vi "aptControl.vi"() -> (0 "Moving":bool, 3 "Current Position":sgl)   [LabVIEW 2014]
uses:
  <vilib>/DAQmx/write.llb/DAQmx Write (Digital 1D Bool 1Chan 1Samp).vi
  <vilib>/DAQmx/write.llb/DAQmx Write (Analog Wfm 1Chan NSamp).vi
  <vilib>/DAQmx/read.llb/DAQmx Read (Analog Wfm 1Chan NSamp).vi
  <vilib>/Analysis/baseanly.llb/Mean (DBL).vi
  <vilib>/DAQmx/miscellaneous.llb/DAQmx Fill In Error Info.vi
  <vilib>/Utility/file.llb/Write To Spreadsheet File (DBL).vi
  <vilib>/Utility/file.llb/Read From Spreadsheet File (DBL).vi
  <vilib>/gmath/NI_Gmath.lvlib
  <vilib>/Analysis/NI_AALBase.lvlib
panel:
  out "Power Min&Max":i32[](array[numeric])
  out "Setup":i32
  out "MirrorPosition":sgl
  out "SavePath":path
  out "MinPos":sgl
  out "MaxPos":sgl
  out "Scaner":string
  in  "Tab Control":enum32{"Control", "Curve", "Calibrate"}(tab)
  in  "Shutter":bool
  in  "Power (mW)":dbl format="%#.0f"
  in  "Possition (0:360)":dbl format="%#.2f"
  in  "Up":bool
  in  "Down":bool
  in  "Mirror\nOverride":bool
  in  "Galvo":bool=TRUE caption="AOD"
  in  "Lens":u16(ring)=10 items=["4X"=4, "10X"=10, "16X"=16, "20X"=20, "25X"=25, "40X"=40, "60X"=60]
  out "Error/Wait":bool
  in  "Home":bool
  in  "stop":bool
  in  "Auto":bool
  out "Calibration Used":string
  out "Curve":cluster{"all rows":dbl[], "all rows":dbl[]}(graph)
  out "Curve 2":cluster{i32[], i32[]}(graph)
  in  "Path":path=path "X:/2Pcalibration"
  in  "Start Calibration":bool
  in  "WaveLengths":dbl[](array[numeric])=[800.0, 890.0]
  out "Finished":bool
  in  "quit":bool
  out "Remaining\n min":dbl format="%#.2f"
  out "Acquiring":bool
  out "Waiting":bool
  out "Moving 2":bool
  in  "Repetitions":dbl=1.0
  in  "Step Size":dbl=4.0
  out "Current mW":dbl format="%#.0f"
  out "Old possition":sgl
  in  "AOD motor":refnum<k7>(container)
  in  "Target Position":dbl
  in  "Attenuator motor":refnum<k7>(container)
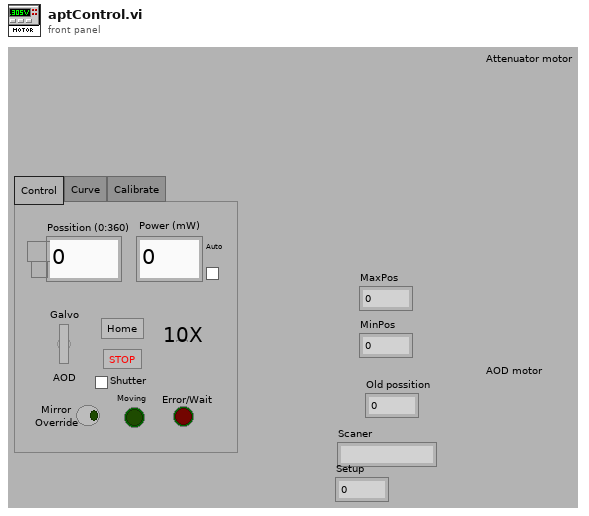
[diagram p1: front panel]
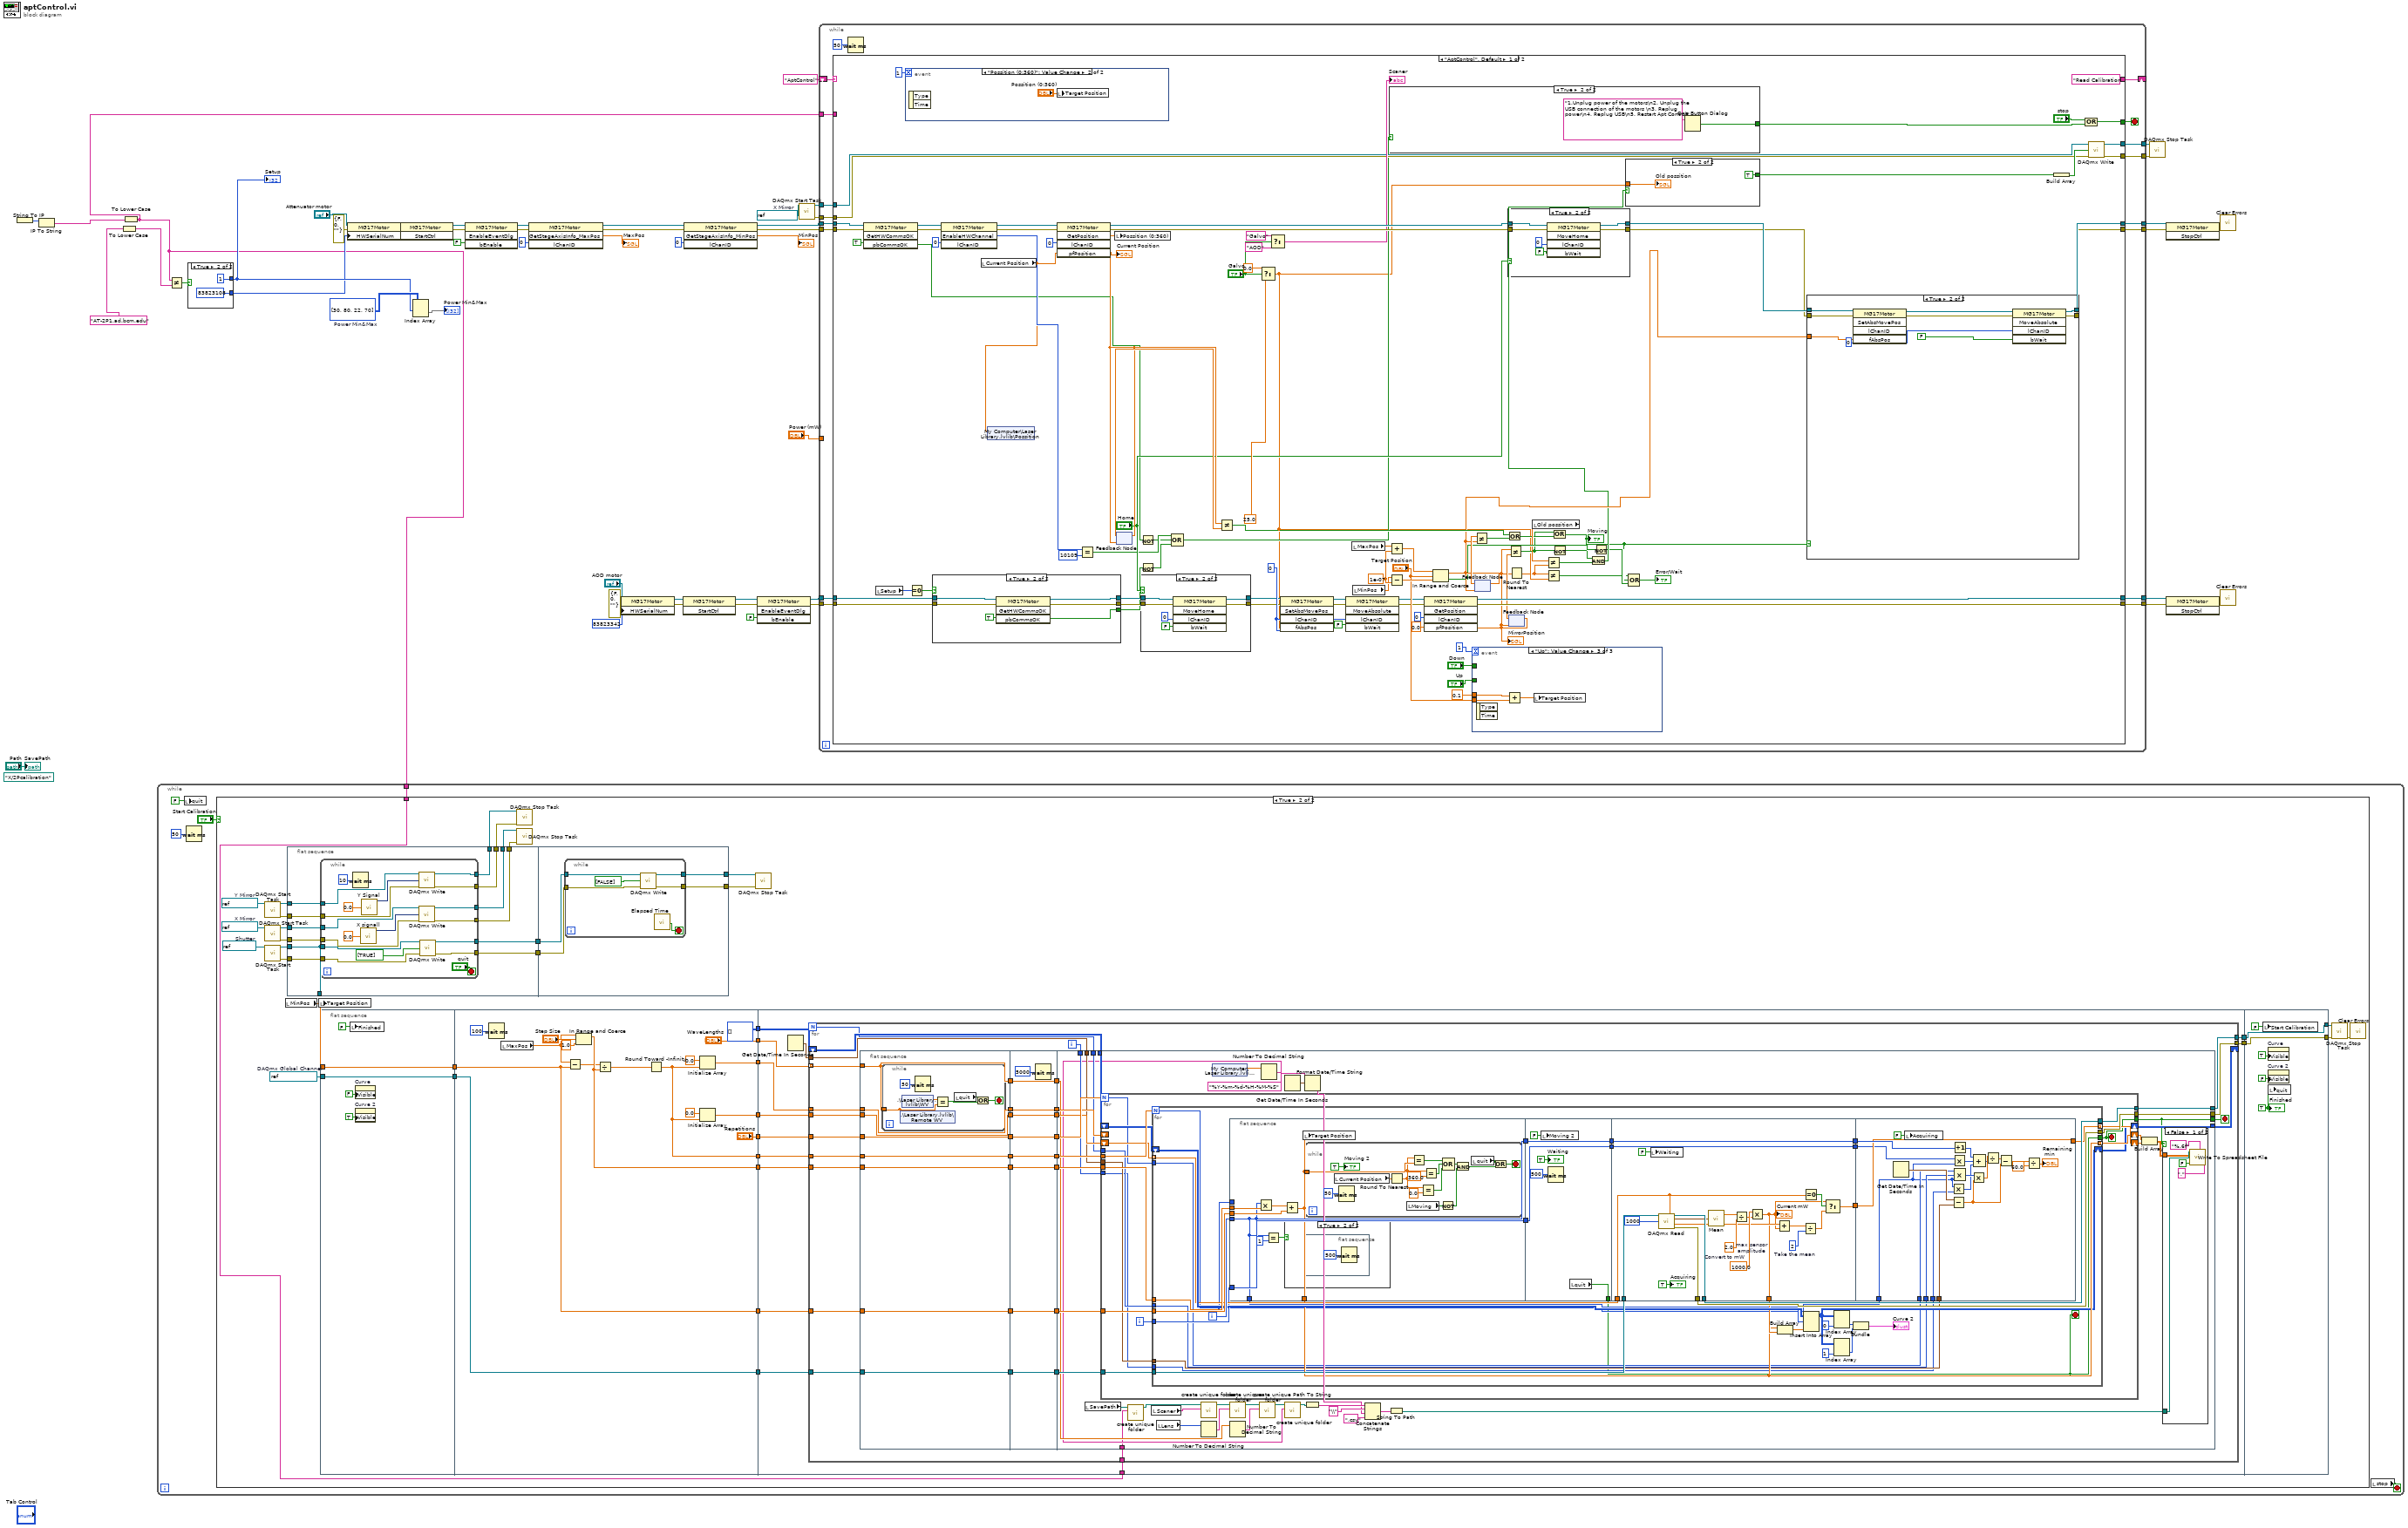
[diagram p0: block diagram]
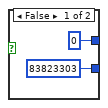
[diagram p2: hidden frame]
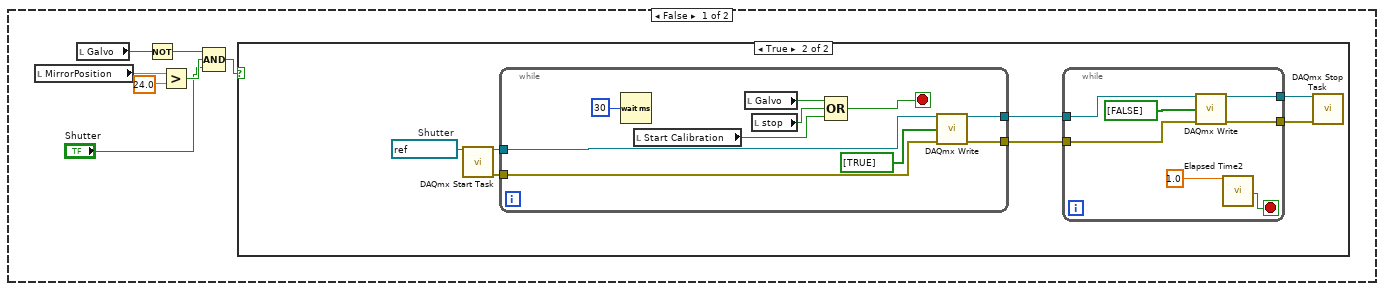
[diagram p3: hidden frame]
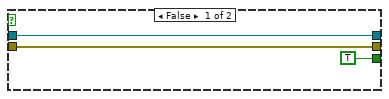
[diagram p7: hidden frame]
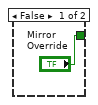
[diagram p9: hidden frame]
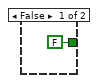
[diagram p10: hidden frame]
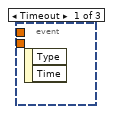
[diagram p11: hidden frame]
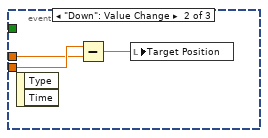
[diagram p12: hidden frame]
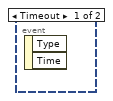
[diagram p13: hidden frame]
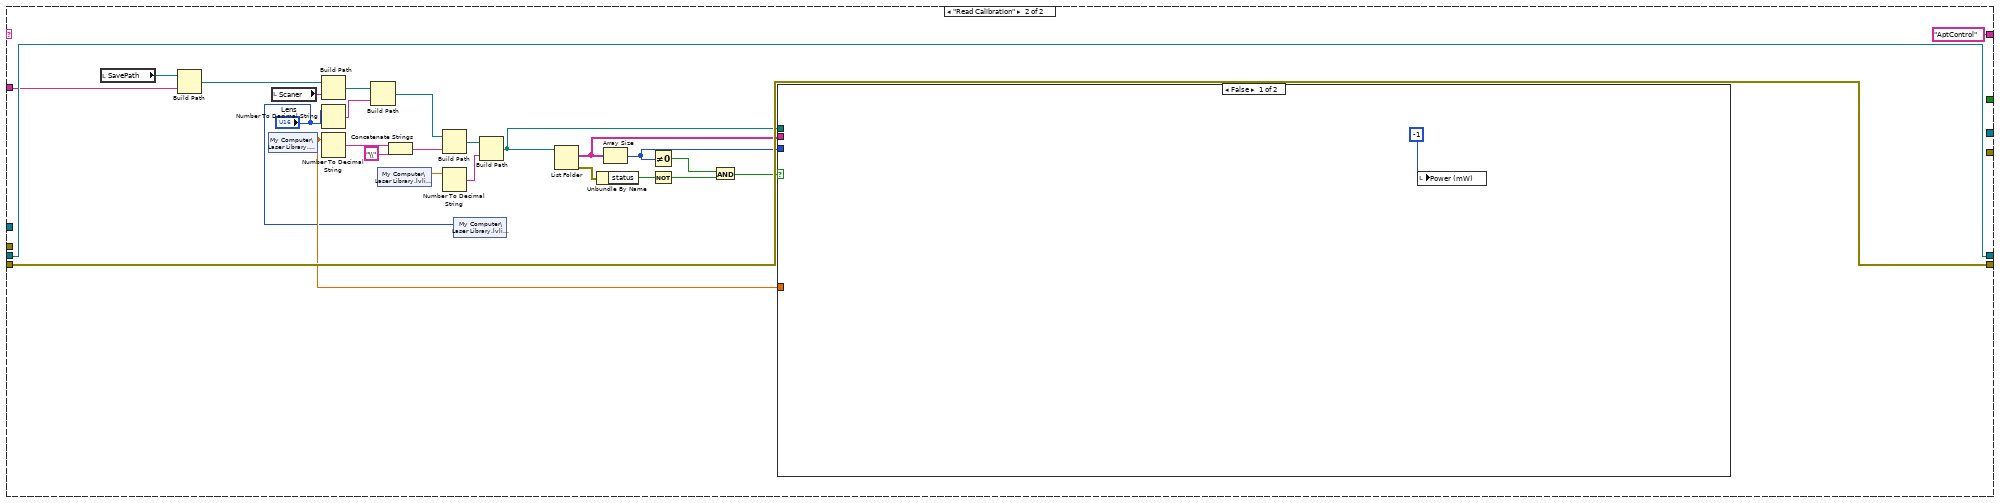
[diagram p16: hidden frame]
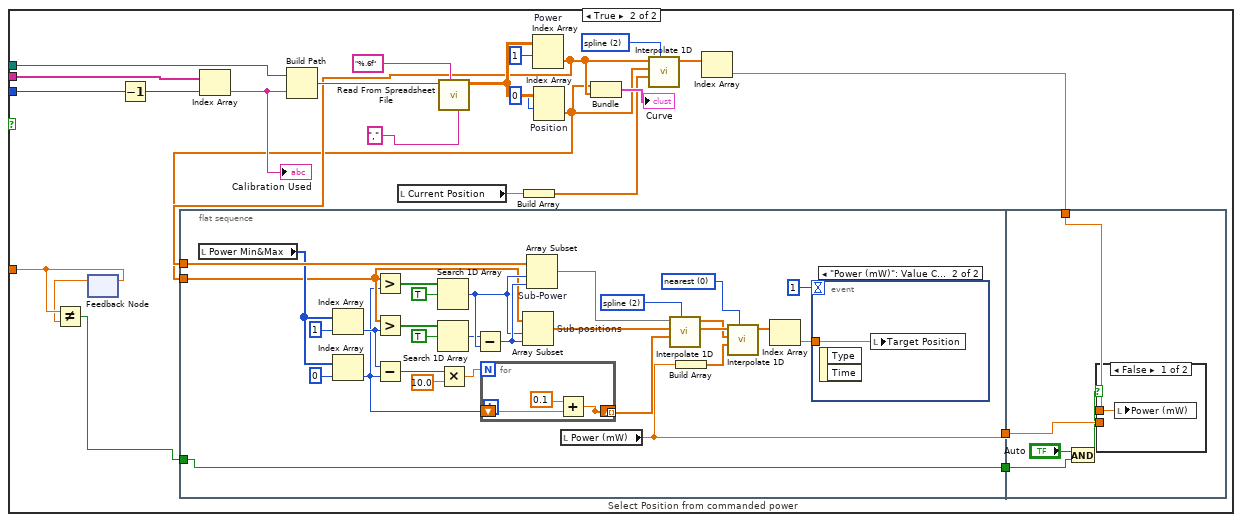
[diagram p17: hidden frame]
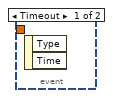
[diagram p18: hidden frame]
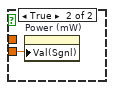
[diagram p19: hidden frame]
diagram:
  w11 = i32[][] [[30, 80], [22, 70]]  # Power Min&Max
  (unwired) path "X:/2Pcalibration"
  w20 = refnum<k21> "FlipMirror"  # X Mirror
  n1 = String To IP() -> (0:w8:u32)  [unwired: 1 in]
  n2 = IP To String(2:w8) -> (0:w4:string)  [unwired: 1 in]
  n3 = To Lower Case(string="AT-2P1.ad.bcm.edu") -> (all lower case string=w2:string)
  n4 = To Lower Case(string=w4) -> (all lower case string=w3:string)
  n5 = while {
    tunnel: w3 -> [w52]
    stop <- w55 stop-if-true
    n6 = local write "quit"(FALSE) -> ()
    n7 = Wait (ms)(milliseconds to wait=u32 50) -> ()  [unwired: 1 out]
    n8 = case shown="True" "Start Calibration" {
      tunnel: w52 -> [_ w88]
      frame False {
        n9 = local read "MirrorPosition"() -> (w63:sgl)
        n10 = local read "Galvo"() -> (w61:bool)
        n11 = Not(x=w61) -> (.not. x?=w62:bool)
        n12 = Greater?(x=w63, y=sgl 24.0) -> (0:w60:bool)
        n13 = Compound Arithmetic op=AND(w62, w60, "Shutter") -> (w58:bool)
        n14 = case shown="True" w58 {
          frame False {
          }
          frame True {
            w70 = refnum<k21> "Shutter"  # Shutter
            n15 = call <vilib>:"DAQmx Start Task.vi"("task/channels in"=w70) -> ("task out"=w69:refnum<k21>, "error out"=w68:errorcluster)  [unwired: 13 in]
            n16 = while {
              tunnel: w69 -> [w86]
              tunnel: w68 -> [w85]
              tunnel: [w84] -> w67
              tunnel: [w83] -> w66
              stop <- w80 stop-if-true
              n17 = Wait (ms)(milliseconds to wait=u32 30) -> ()  [unwired: 1 out]
              n18 = local read "Start Calibration"() -> (w81:bool)
              n19 = local read "Galvo"() -> (w78:bool)
              n20 = local read "stop"() -> (w82:bool)
              n21 = Compound Arithmetic op=OR(w78, w82, w81) -> (w80:bool)
              n22 = call-poly <vilib>:"DAQmx Write.vi"("task/channels in"=w86, "data"=bool[] [TRUE], "error in"=w85) -> ("task out"=w84:refnum<k21>, "error out"=w83:errorcluster)  [unwired: 10 in, 1 out]
            }
            n23 = while {
              tunnel: w67 -> [w77]
              tunnel: w66 -> [w76]
              tunnel: [w75] -> w65
              tunnel: [w74] -> w64
              stop <- w72 stop-if-true
              n24 = call-poly <vilib>:"DAQmx Write.vi"("task/channels in"=w77, "data"=bool[] [FALSE], "error in"=w76) -> ("task out"=w75:refnum<k21>, "error out"=w74:errorcluster)  [unwired: 10 in, 1 out]
              n25 = call "Elapsed Time2"("Time Target (s)"=1.0) -> ("Time has Elapsed"=w72:bool)  [unwired: 11 in, 7 out]
            }
            n26 = call <vilib>:"DAQmx Stop Task.vi"("task/channels in"=w65, "error in"=w64) -> ()  [unwired: 12 in, 2 out]
          }
        }
      }
      frame True {
        w96 = refnum<k21> "Y Mirror"  # Y Mirror
        w97 = refnum<k21> "X Mirror"  # X Mirror
        w98 = refnum<k21> "Shutter"  # Shutter
        w105 = refnum<k21> "PowerMeter"  # DAQmx Global Channel
        n27 = call <vilib>:"DAQmx Start Task.vi"("task/channels in"=w96) -> ("task out"=w95:refnum<k21>, "error out"=w90:errorcluster)  [unwired: 13 in]
        n28 = call <vilib>:"DAQmx Start Task.vi"("task/channels in"=w97) -> ("task out"=w93:refnum<k21>, "error out"=w91:errorcluster)  [unwired: 13 in]
        n29 = call <vilib>:"DAQmx Start Task.vi"("task/channels in"=w98) -> ("task out"=w94:refnum<k21>, "error out"=w92:errorcluster)  [unwired: 13 in]
        n30 = local read "MinPos"() -> (w89:sgl)
        n31 = flat-sequence {
          tunnel: [w127] -> _
          tunnel: w93 -> [w135]
          tunnel: [w134] -> w110
          tunnel: [w133] -> w109
          tunnel: [w132] -> w102
          tunnel: [w131] -> w101
          tunnel: [w130] -> w100
          tunnel: [w129] -> w99
          tunnel: w95 -> [w128]
          tunnel: w94 -> [w127]
          tunnel: w92 -> [w126]
          tunnel: w91 -> [w125]
          tunnel: w90 -> [w124]
          tunnel: w110 -> [w158]
          tunnel: [w157] -> w104
          tunnel: [w156] -> w103
          tunnel: w109 -> [w155]
          frame #0 {
            n32 = while {
              tunnel: w127 -> [w149]
              tunnel: w135 -> [w151]
              tunnel: w128 -> [w150]
              tunnel: [w147] -> w134
              tunnel: [w146] -> w133
              tunnel: [w143] -> w132
              tunnel: [w142] -> w131
              tunnel: [w141] -> w130
              tunnel: [w140] -> w129
              tunnel: w126 -> [w139]
              tunnel: w125 -> [w138]
              tunnel: w124 -> [w137]
              stop <- "quit" stop-if-true
              n33 = Wait (ms)(milliseconds to wait=u32 10) -> ()  [unwired: 1 out]
              n34 = call "X signall"("Amplitude"=0.0) -> ("Sine"=w145:dynamicdata)  [unwired: 13 in, 1 out]
              n35 = call "Y Signal"("Amplitude"=0.0) -> ("Sine"=w144:dynamicdata)  [unwired: 13 in, 1 out]
              n36 = call-poly <vilib>:"DAQmx Write.vi"("task/channels in"=w150, "data"=w144, "error in"=w137) -> ("task out"=w141:refnum<k21>, "error out"=w140:errorcluster)  [unwired: 10 in, 1 out]
              n37 = call-poly <vilib>:"DAQmx Write.vi"("task/channels in"=w151, "data"=w145, "error in"=w138) -> ("task out"=w143:refnum<k21>, "error out"=w142:errorcluster)  [unwired: 10 in, 1 out]
              n38 = call-poly <vilib>:"DAQmx Write.vi"("task/channels in"=w149, "data"=bool[] [TRUE], "error in"=w139) -> ("task out"=w147:refnum<k21>, "error out"=w146:errorcluster)  [unwired: 10 in, 1 out]
            }
          }
          frame #1 {
            n39 = while {
              tunnel: w158 -> [w163]
              tunnel: [w161] -> w157
              tunnel: [w160] -> w156
              tunnel: w155 -> [w159]
              stop <- w164 stop-if-true
              n40 = call-poly <vilib>:"DAQmx Write.vi"("task/channels in"=w163, "data"=bool[] [FALSE], "error in"=w159) -> ("task out"=w161:refnum<k21>, "error out"=w160:errorcluster)  [unwired: 10 in, 1 out]
              n41 = call "Elapsed Time"() -> ("Time has Elapsed"=w164:bool)  [unwired: 12 in, 7 out]
            }
          }
        }
        n42 = local write "Target Position"(w89) -> ()
        n43 = flat-sequence {
          tunnel: w105 -> [w168]
          tunnel: w89 -> [w169]
          tunnel: [w169] -> w123
          tunnel: [w168] -> w122
          tunnel: [w184] -> w121
          tunnel: ["Repetitions"] -> w120
          tunnel: [w183] -> w119
          tunnel: [w186] -> w118
          tunnel: [w182] -> w117
          tunnel: [w181] -> w116
          tunnel: [i32[][] []] -> w115
          tunnel: ["WaveLengths"] -> w114
          tunnel: [w180] -> w113
          tunnel: w123 -> [w184]
          tunnel: w122 -> [w186]
          tunnel: w121 -> [w199]
          tunnel: w120 -> [w198]
          tunnel: w119 -> [w197]
          tunnel: w118 -> [w196]
          tunnel: w117 -> [w194]
          tunnel: w116 -> [w193]
          tunnel: w115 -> [w191]
          tunnel: w114 -> [w192]
          tunnel: w113 -> [w195]
          tunnel: [w190] -> w112
          tunnel: [w189] -> w111
          tunnel: w88 -> [w187]
          tunnel: [w427] -> w106
          tunnel: [w428] -> w107
          tunnel: w112 -> [w428]
          tunnel: w111 -> [w427]
          frame #0 {
            n44 = local write "Finished"(FALSE ("Finished")) -> ()
            n45 = property on="Curve" class="XYGraph (strict)"("Visible"=FALSE) -> ()  [unwired: 2 in, 2 out]
            n46 = property on="Curve 2" class="XYGraph (strict)"("Visible"=TRUE) -> ()  [unwired: 2 in, 2 out]
          }
          frame #1 {
            n47 = Wait (ms)(milliseconds to wait=u32 100) -> ()  [unwired: 1 out]
            n48 = local read "MaxPos"() -> (w170:sgl)
            n49 = Subtract(x=w170, y=w184) -> (x-y=w175:sgl)
            n50 = In Range and Coerce(upper limit=w170, x="Step Size", lower limit=1.0) -> (coerced(x)=w183:dbl)  [unwired: 1 out]
            n51 = Divide(x=w175, y=w183) -> (x/y=w176:dbl)
            n52 = Round Toward -Infinity(1:w176) -> (0:w182:dbl)
            n53 = Initialize Array(0.0 ("element"), w182) -> (w181:dbl[])
            n54 = Initialize Array(0.0 ("element"), w182) -> (w180:dbl[])
          }
          frame #2 {
            n55 = Get Date/Time In Seconds() -> (seconds since 1Jan1904=w188:timestamp)
            n56 = for {
              N -> [w203]
              tunnel: w199 -> [w232]
              tunnel: w198 -> [w231]
              tunnel: w197 -> [w230]
              tunnel: w196 -> [w229]
              tunnel: [w228] -> w190
              tunnel: [w227] -> w189
              tunnel: w195 -> [w226]
              tunnel: w194 -> [w225]
              tunnel: w193 -> [w224]
              tunnel: w192 -> [w223] mode=indexing
              shift-right: [w205] -> _
              shift-left: w191 -> [w206]
              tunnel: w188 -> [w204]
              tunnel: w187 -> [w200]
              i -> [w202]
              stop <- w201 stop-if-true
              n57 = flat-sequence {
                tunnel: w223 -> [w233]
                tunnel: w224 -> [w234]
                tunnel: w225 -> [w235]
                tunnel: w226 -> [w236]
                tunnel: w229 -> [w237]
                tunnel: w230 -> [w238]
                tunnel: w231 -> [w239]
                tunnel: w232 -> [w240]
                tunnel: [w240] -> w222
                tunnel: [w239] -> w220
                tunnel: [w238] -> w218
                tunnel: [w237] -> w216
                tunnel: [w236] -> w214
                tunnel: [w235] -> w212
                tunnel: [w234] -> w210
                tunnel: [w233] -> w208
                tunnel: w222 -> [w255]
                tunnel: [w255] -> w221
                tunnel: w220 -> [w254]
                tunnel: [w254] -> w219
                tunnel: w218 -> [w253]
                tunnel: [w253] -> w217
                tunnel: w216 -> [w252]
                tunnel: [w252] -> w215
                tunnel: w214 -> [w251]
                tunnel: [w251] -> w213
                tunnel: w212 -> [w250]
                tunnel: [w250] -> w211
                tunnel: w210 -> [w249]
                tunnel: [w249] -> w209
                tunnel: w208 -> [w248]
                tunnel: [w248] -> w207
                tunnel: [w293] -> w205
                tunnel: [w294] -> w227
                tunnel: [w295] -> w228
                tunnel: w202 -> [w267]
                tunnel: w203 -> [w268]
                tunnel: w204 -> [w269]
                tunnel: w206 -> [w270]
                tunnel: w207 -> [w271]
                tunnel: w209 -> [w286]
                tunnel: w211 -> [w287]
                tunnel: w213 -> [w288]
                tunnel: w215 -> [w289]
                tunnel: w217 -> [w290]
                tunnel: w219 -> [w291]
                tunnel: w221 -> [w292]
                tunnel: [w258] -> w201
                tunnel: w200 -> [w256]
                frame #0 {
                  n58 = while {
                    tunnel: w233 -> [w245]
                    stop <- w241 stop-if-true
                    n59 = shared-variable ".\\Laser Library.lvlib\\Remote WV"(w245) -> ()  [unwired: 1 in, 1 out]
                    n60 = shared-variable ".\\Laser Library.lvlib\\WV"() -> (w244:dbl)  [unwired: 1 in, 1 out]
                    n61 = Wait (ms)(milliseconds to wait=u32 50) -> ()  [unwired: 1 out]
                    n62 = Equal?(x=w244, y=w245) -> (x = y?=w242:bool)
                    n63 = local read "quit"() -> (w243:bool)
                    n64 = Or(x=w243, y=w242) -> (x .or. y?=w241:bool)
                  }
                }
                frame #1 {
                  n65 = Wait (ms)(milliseconds to wait=u32 5000) -> ()  [unwired: 1 out]
                }
                frame #2 {
                  n66 = local read "SavePath"() -> (w257:path)
                  n67 = for {
                    N: w291 -> [w303]
                    tunnel: w287 -> [w317]
                    tunnel: w292 -> [w316]
                    tunnel: w290 -> [w315]
                    tunnel: w289 -> [w314]
                    tunnel: [w313] -> w295
                    tunnel: [w312] -> w294
                    shift-right: [w311] -> w273
                    shift-left: w288 -> [w309]
                    shift-right: [w310] -> w274
                    shift-left: w286 -> [_]
                    shift-right: [w308] -> w293
                    shift-left: w270 -> [w307]
                    tunnel: w269 -> [w305]
                    tunnel: w268 -> [w304]
                    tunnel: w267 -> [w302]
                    tunnel: [w301] -> w258
                    i -> [w306]
                    stop <- w301 stop-if-true
                    n68 = for {
                      N: w317 -> [w321]
                      tunnel: w316 -> [w350]
                      tunnel: w315 -> [w349]
                      tunnel: w314 -> [w347]
                      tunnel: [w346] -> w313
                      tunnel: [w345] -> w312
                      tunnel: [w320] -> w311 mode=indexing
                      tunnel: w309 -> [w342] mode=indexing
                      tunnel: [w338] -> w310 mode=indexing
                      shift-right: [w335] -> w308
                      shift-left: w307 -> [w343]
                      tunnel: w306 -> [w332]
                      tunnel: w305 -> [w331]
                      tunnel: w304 -> [w330]
                      tunnel: w303 -> [w329]
                      tunnel: w302 -> [w328]
                      tunnel: [w319] -> w301
                      i -> [w348]
                      stop <- w319 stop-if-true
                      n69 = flat-sequence {
                        tunnel: w348 -> [w354]
                        tunnel: w349 -> [w358]
                        tunnel: w350 -> [w355]
                        tunnel: [w351] -> w338
                        tunnel: [w354] -> w339
                        tunnel: w332 -> [w357]
                        tunnel: [w357] -> w325
                        tunnel: [w354] -> w322
                        tunnel: w321 -> [_]
                        tunnel: [w380] -> w326
                        tunnel: w325 -> [w380]
                        tunnel: [w379] -> w323
                        tunnel: w322 -> [w379]
                        tunnel: [w376] -> w319
                        tunnel: w347 -> [w401]
                        tunnel: [w400] -> w346
                        tunnel: [w399] -> w345
                        tunnel: w342 -> [w385]
                        tunnel: [w393] -> w344
                        tunnel: [w382] -> w341
                        tunnel: [w387] -> w327
                        tunnel: w326 -> [w387]
                        tunnel: [w386] -> w324
                        tunnel: w323 -> [w386]
                        tunnel: w344 -> [w416]
                        tunnel: w331 -> [w421]
                        tunnel: w330 -> [w420]
                        tunnel: w329 -> [w419]
                        tunnel: w321 -> [w408]
                        tunnel: w328 -> [w409]
                        tunnel: w327 -> [w410]
                        tunnel: w324 -> [w418]
                        tunnel: [w416] -> w320
                        frame #0 {
                          n70 = Multiply(x=w354, y=w358) -> (x*y=w356:dbl)
                          n71 = Equal?(x=w354, y=1) -> (x = y?=w353:bool)
                          n72 = Add(x=w356, y=w355) -> (x+y=w351:dbl)
                          n73 = case shown="True" w353 {
                            frame False {
                            }
                            frame True {
                              n74 = flat-sequence {
                                frame #0 {
                                n75 = Wait (ms)(milliseconds to wait=u32 500) -> ()  [unwired: 1 out]
                                }
                              }
                            }
                          }
                          n76 = local write "Target Position"(w351) -> ()
                          n77 = while {
                            tunnel: w351 -> [w374]
                            stop <- w361 stop-if-true
                            n78 = local read "Current Position"() -> (w363:sgl)
                            n79 = Wait (ms)(milliseconds to wait=u32 50) -> ()  [unwired: 1 out]
                            n80 = Round To Nearest(number=w363) -> (nearest integer value=w368:sgl)
                            n81 = local read "Moving"() -> (w364:bool)
                            n82 = Equal?(x=w368, y=w374) -> (x = y?=w372:bool)
                            n83 = Equal?(x=w368, y=0.0) -> (x = y?=w369:bool)
                            n84 = Equal?(x=w368, y=360.0) -> (x = y?=w370:bool)
                            n85 = Not(x=w364) -> (.not. x?=w373:bool)
                            n86 = Compound Arithmetic op=OR(w372, w370, w369) -> (w371:bool)
                            n87 = And(x=w371, y=w373) -> (x .and. y?=w362:bool)
                            n88 = local read "quit"() -> (w360:bool)
                            n89 = Or(x=w360, y=w362) -> (x .or. y?=w361:bool)
                            "Moving 2" <- TRUE
                          }
                        }
                        frame #1 {
                          n90 = local write "Moving 2"(FALSE) -> ()
                          n91 = Wait (ms)(milliseconds to wait=u32 500) -> ()  [unwired: 1 out]
                          n92 = local read "quit"() -> (w376:bool)
                          "Waiting" <- TRUE
                        }
                        frame #2 {
                          w388 = 2.0  # max sensor  amplitude
                          w390 = 1000.0  # Convert to mW
                          w396 = 2  # Take the mean
                          n93 = local write "Waiting"(FALSE) -> ()
                          n94 = call-poly <vilib>:"DAQmx Read.vi"("task/channels in"=w401, "number of samples per channel"=1000) -> ("task out"=w400:refnum<k21>, "data"=w391:waveform(dbl), "error out"=w399:errorcluster)  [unwired: 1 in, 10 out]
                          n95 = call-poly <vilib>:"Mean.vi"("X"=w391) -> ("mean"=w392:dbl)  [unwired: 1 out]
                          n96 = Divide(x=w392, y=w388) -> (x/y=w389:dbl)
                          n97 = Multiply(x=w390, y=w389) -> (x*y=w382:dbl)
                          "Current mW" <- w382
                          n98 = Add(x=w385, y=w382) -> (x+y=w395:dbl)
                          n99 = Divide(x=w395, y=w396) -> (x/y=w394:dbl)
                          n100 = Equal To 0?(x=w385) -> (x = 0?=w397:bool)
                          n101 = Select(t=w382, s=w397, f=w394) -> (s? t:f=w393:dbl)
                          "Acquiring" <- TRUE ("Acquiring")
                        }
                        frame #3 {
                          n102 = Get Date/Time In Seconds() -> (seconds since 1Jan1904=w422:timestamp)
                          n103 = local write "Acquiring"(FALSE ("Acquiring")) -> ()
                          n104 = Multiply(x=w408, y=w409) -> (x*y=w405:i32)
                          n105 = Subtract(x=w422, y=w421) -> (x-y=w413:dbl)
                          n106 = Multiply(x=w410, y=w408) -> (x*y=w406:i32)
                          n107 = Increment(x=w418) -> (x+1=w407:i32)
                          n108 = Compound Arithmetic op=MULTIPLY(w419, w420, w408) -> (w415:i32)
                          n109 = Multiply(x=w415, y=w413) -> (x*y=w414:dbl)
                          n110 = Compound Arithmetic op=ADD(w407, w406, w405) -> (w404:i32)
                          n111 = Divide(x=w414, y=w404) -> (x/y=w412:dbl)
                          n112 = Subtract(x=w412, y=w413) -> (x-y=w411:dbl)
                          n113 = Divide(x=w411, y=60.0) -> (x/y=→"Remaining\n min":dbl)
                        }
                      }
                      n114 = Build Array(w338, w341) -> (w340:dbl[])
                      n115 = Insert Into Array(array=w343, index (row)=w339, new element=w340) -> (w335:i32[][])  [unwired: 1 in]
                      n116 = Index Array(array=w335, index (col)=0 ("index")) -> (element=w336:i32[])  [unwired: 1 in]
                      n117 = Index Array(array=w335, index (col)=1 ("index")) -> (element=w333:i32[])  [unwired: 1 in]
                      n118 = Bundle(w336, w333) -> (→"Curve 2":cluster{i32[], i32[]})  [unwired: 1 in]
                    }
                  }
                  n119 = call "create unique folder.vi"("string"=w256, "path 2"=w257) -> ("path"=w266:path)  [unwired: 9 in]
                  n120 = local read "Scaner"() -> (w259:string)
                  n121 = local read "Lens"() -> (w260:u16)
                  n122 = call "create unique folder.vi"("string"=w259, "path 2"=w266) -> ("path"=w265:path)  [unwired: 9 in]
                  n123 = Number To Decimal String(number=w260) -> (decimal integer string=w275:string)  [unwired: 1 in]
                  n124 = shared-variable "My Computer\\Laser Library.lvlib\\GDD"() -> (w264:dbl)  [unwired: 1 in, 1 out]
                  n125 = call "create unique folder.vi"("string"=w275, "path 2"=w265) -> ("path"=w276:path)  [unwired: 9 in]
                  n126 = Number To Decimal String(number=w271) -> (decimal integer string=w283:string)  [unwired: 1 in]
                  n127 = call "create unique folder.vi"("string"=w283, "path 2"=w276) -> ("path"=w263:path)  [unwired: 9 in]
                  n128 = Number To Decimal String(number=w264) -> (decimal integer string=w261:string)  [unwired: 1 in]
                  n129 = Get Date/Time In Seconds() -> (seconds since 1Jan1904=w285:timestamp)
                  n130 = call "create unique folder.vi"("string"=w261, "path 2"=w263) -> ("path"=w262:path)  [unwired: 9 in]
                  n131 = Path To String(path=w262) -> (string=w282:string)
                  n132 = Format Date/Time String(time format string (%c)="%Y-%m-%d-%H-%M-%S", seconds (now)=w285) -> (date/time string=w280:string)  [unwired: 1 in]
                  n133 = Concatenate Strings(w282, "\\" ("string"), w280, ".csv" ("string")) -> (w279:string)
                  n134 = String To Path(string=w279) -> (path=w278:path)
                  n135 = Build Array(w274, w273) -> (w272:dbl[][])
                  n136 = case shown="False" w258 {
                    tunnel: w278 -> [w297 _]
                    tunnel: w272 -> [w296 _]
                    frame False {
                      n137 = call-poly <vilib>:"Write To Spreadsheet File.vi"("delimiter (\\t)"="," ("delimiter (\\t)"), "format (%.3f)"="%.6f", "append to file? (new file:F)"=FALSE, "2D data"=w296, "file path (dialog if empty)"=w297) -> ()  [unwired: 2 in, 2 out]
                    }
                    frame True {
                    }
                  }
                }
              }
            }
          }
          frame #3 {
            w426 = TRUE ("Finished")
            n138 = local write "Start Calibration"(FALSE) -> ()
            n139 = property on="Curve" class="XYGraph (strict)"("Visible"=TRUE) -> ()  [unwired: 2 in, 2 out]
            n140 = property on="Curve 2" class="XYGraph (strict)"("Visible"=FALSE) -> ()  [unwired: 2 in, 2 out]
            n141 = local write "quit"(w426) -> ()
            "Finished" <- w426
          }
        }
        n142 = call <vilib>:"DAQmx Stop Task.vi"("task/channels in"=w100, "error in"=w99) -> ()  [unwired: 12 in, 2 out]
        n143 = call <vilib>:"DAQmx Stop Task.vi"("task/channels in"=w102, "error in"=w101) -> ()  [unwired: 12 in, 2 out]
        n144 = call <vilib>:"DAQmx Stop Task.vi"("task/channels in"=w104, "error in"=w103) -> ()  [unwired: 12 in, 2 out]
        n145 = call <vilib>:"DAQmx Stop Task.vi"("task/channels in"=w107, "error in"=w106) -> ("error out"=w108:errorcluster)  [unwired: 13 out]
        n146 = call <vilib>:"Clear Errors.vi"("error in (no error)"=w108) -> ()  [unwired: 5 in, 2 out]
      }
    }
    n147 = local read "stop"() -> (w55:bool)
  }
  n148 = Not Equal?(x=w3, y=w2) -> (x != y?=w7:bool)
  n149 = case shown="True" w7 {
    tunnel: [0 1] -> w6
    tunnel: [83823303 83823108] -> w5
    frame False {
    }
    frame True {
    }
  }
  "Setup" <- w6
  n150 = property class="MG17Motor"(reference="Attenuator motor", error in=errorcluster {"status"=FALSE, "code"=0, "source"=""} ("error in (no error)"), "HWSerialNum"=w5) -> (reference out=w50:refnum<k7>, error out=w49:errorcluster)
  n151 = invoke class="MG17Motor" method="StartCtrl"(reference=w50, error in=w49) -> (reference out=w38:refnum<k7>, error out=w37:errorcluster)  [unwired: 1 in, 1 out]
  n152 = Index Array(array=w11, index (row)=w6) -> (element=→"Power Min&Max":i32[])  [unwired: 1 in]
  n153 = invoke class="MG17Motor" method="EnableEventDlg"(reference=w38, error in=w37, "bEnable"=FALSE) -> (reference out=w36:refnum<k7>, error out=w35:errorcluster)  [unwired: 1 in, 2 out]
  n154 = invoke class="MG17Motor" method="GetStageAxisInfo_MaxPos"(reference=w36, error in=w35, "lChanID"=0) -> (reference out=w41:refnum<k7>, error out=w40:errorcluster, "GetStageAxisInfo_MaxPos"=→"MaxPos":sgl)  [unwired: 1 in, 1 out]
  n155 = property class="MG17Motor"(reference="AOD motor", error in=errorcluster {"status"=FALSE, "code"=0, "source"=""} ("error in (no error)"), "HWSerialNum"=83823342) -> (reference out=w30:refnum<k7>, error out=w31:errorcluster)
  n156 = invoke class="MG17Motor" method="StartCtrl"(reference=w30, error in=w31) -> (reference out=w33:refnum<k7>, error out=w34:errorcluster)  [unwired: 1 in, 1 out]
  n157 = invoke class="MG17Motor" method="GetStageAxisInfo_MinPos"(reference=w41, error in=w40, "lChanID"=0) -> (reference out=w48:refnum<k7>, error out=w43:errorcluster, "GetStageAxisInfo_MinPos"=→"MinPos":sgl)  [unwired: 1 in, 1 out]
  n158 = invoke class="MG17Motor" method="EnableEventDlg"(reference=w33, error in=w34, "bEnable"=FALSE) -> (reference out=w28:refnum<k7>, error out=w23:errorcluster)  [unwired: 1 in, 2 out]
  n159 = call <vilib>:"DAQmx Start Task.vi"("task/channels in"=w20) -> ("task out"=w17:refnum<k21>, "error out"=w16:errorcluster)  [unwired: 13 in]
  n160 = while {
    tunnel: w48 -> [w449]
    tunnel: [w446] -> w46
    tunnel: [w447] -> w45
    tunnel: w43 -> [w445]
    shift-right: [w442] -> _
    shift-left: "AptControl" -> [w443]
    tunnel: w3 -> [w441]
    tunnel: w28 -> [w440]
    tunnel: [w439] -> w25
    tunnel: [w438] -> w24
    tunnel: w23 -> [w437]
    tunnel: [w436] -> w19
    tunnel: [w435] -> w18
    tunnel: w17 -> [w434]
    tunnel: w16 -> [w433]
    tunnel: "Power (mW)" -> [_]
    stop <- w444 stop-if-true
    n161 = case shown="\"AptControl\", Default" w443 {
      tunnel: w449 -> [w475 w614]
      tunnel: [w530 w614] -> w447
      tunnel: [w529 w613] -> w446
      tunnel: w445 -> [w473 w613]
      tunnel: [w523 _] -> w444
      tunnel: ["Read Calibration" "AptControl"] -> w442
      tunnel: w441 -> [_ w610]
      tunnel: w440 -> [w471 _]
      tunnel: [w501 _] -> w439
      tunnel: [w500 _] -> w438
      tunnel: w437 -> [w469 _]
      tunnel: [w482 _] -> w436
      tunnel: [w481 _] -> w435
      tunnel: w434 -> [w480 _]
      tunnel: w433 -> [w479 _]
      frame "AptControl", Default {
        w509 = 0 ("lChanID")
        w532 = 1e-07
        n162 = invoke class="MG17Motor" method="GetHWCommsOK"(reference=w475, error in=w473, "pbCommsOK"=TRUE) -> (reference out=w474:refnum<k7>, error out=w472:errorcluster, "pbCommsOK"=w463:bool)  [unwired: 1 in, 1 out]
        n163 = local read "Setup"() -> (w452:i32)
        n164 = event shown="[1] \"Possition (0:360)\": Value Change" {
          selector: _ -> [_ _]
          dyn-events: _ -> [_ _]
          timeout: 1 -> [_ _]
          event Timeout {
            n165 = event-data() -> ()  [unwired: 1 in, 2 out]
          }
          event "Possition (0:360)": Value Change {
            n166 = event-data() -> ()  [unwired: 1 in, 2 out]
            n167 = local write "Target Position"("Possition (0:360)") -> ()
          }
        }
        n168 = Equal To 0?(x=w452) -> (x = 0?=w451:bool)
        n169 = case shown="True" w451 {
          tunnel: w471 -> [w543 w548]
          tunnel: [w543 w547] -> w470
          tunnel: w469 -> [w542 w546]
          tunnel: [w542 w545] -> w468
          tunnel: [TRUE ("pbCommsOK") w544] -> w461
          frame False {
          }
          frame True {
            n170 = invoke class="MG17Motor" method="GetHWCommsOK"(reference=w548, error in=w546, "pbCommsOK"=TRUE) -> (reference out=w547:refnum<k7>, error out=w545:errorcluster, "pbCommsOK"=w544:bool)  [unwired: 1 in, 1 out]
          }
        }
        n171 = invoke class="MG17Motor" method="EnableHWChannel"(reference=w474, error in=w472, "lChanID"=0) -> (reference out=w513:refnum<k7>, error out=w512:errorcluster, "EnableHWChannel"=w511:i32)  [unwired: 1 in, 1 out]
        n172 = local read "Current Position"() -> (w450:sgl)
        n173 = shared-variable "My Computer\\Laser Library.lvlib\\Possition"(w450) -> ()  [unwired: 1 in, 1 out]
        n174 = invoke class="MG17Motor" method="GetPosition"(reference=w513, error in=w512, "lChanID"=0, "pfPosition"=w450) -> (reference out=w528:refnum<k7>, error out=w515:errorcluster, "pfPosition"=w522:sgl)  [unwired: 1 in, 2 out]
        "Current Position" <- w522
        n175 = Equal?(x=w511, y=10109) -> (x = y?=w467:bool)
        n176 = local write "Possition (0:360)"(w522) -> ()
        n177 = feedback #1(w522) -> (w537:sgl)
        n178 = feedback-in #1(w522) -> ()
        n179 = Not(x=w463) -> (.not. x?=w462:bool)
        n180 = Not(x=w461) -> (.not. x?=w460:bool)
        n181 = case shown="True" "Home" {
          tunnel: [w550 w555] -> w488
          tunnel: [w551 w554] -> w487
          tunnel: w470 -> [w550 w553]
          tunnel: w468 -> [w551 w552]
          frame False {
          }
          frame True {
            n182 = invoke class="MG17Motor" method="MoveHome"(reference=w553, error in=w552, "lChanID"=0, "bWait"=FALSE) -> (reference out=w555:refnum<k7>, error out=w554:errorcluster)  [unwired: 1 in, 3 out]
          }
        }
        n183 = Compound Arithmetic op=OR(w467, w462, w460) -> (w466:bool)
        n184 = Not Equal?(x=w522, y=w537) -> (x != y?=w536:bool)
        n185 = Select(t=sgl 0.0 ("pfPosition"), s="Galvo", f=sgl 25.0 ("pfPosition")) -> (s? t:f=w457:sgl)
        n186 = Select(t="Galvo", s="Galvo", f="AOD") -> (s? t:f=→"Scaner":string)
        n187 = invoke class="MG17Motor" method="SetAbsMovePos"(reference=w488, error in=w487, "lChanID"=w509, "fAbsPos"=w457) -> (reference out=w507:refnum<k7>, error out=w510:errorcluster)  [unwired: 1 in, 3 out]
        n188 = invoke class="MG17Motor" method="MoveAbsolute"(reference=w507, error in=w510, "lChanID"=w509, "bWait"=FALSE) -> (reference out=w503:refnum<k7>, error out=w502:errorcluster)  [unwired: 1 in, 3 out]
        n189 = local read "MaxPos"() -> (w465:sgl)
        n190 = local read "MinPos"() -> (w464:sgl)
        n191 = case shown="True" w466 {
          tunnel: [FALSE ("true") w562] -> w453
          frame False {
          }
          frame True {
            n192 = One Button Dialog(message="1.Unplug power of the motors\n2. Unplug the USB connection of the motors \n3. Replug power\n4. Replug USB\n5. Restart Apt Control") -> (true=w562:bool)  [unwired: 1 in]
          }
        }
        n193 = Add(x=w465, y=w532) -> (x+y=w533:dbl)
        n194 = Subtract(x=w464, y=w532) -> (x-y=w531:dbl)
        n195 = invoke class="MG17Motor" method="GetPosition"(reference=w503, error in=w502, "lChanID"=0, "pfPosition"=sgl 0.0) -> (reference out=w501:refnum<k7>, error out=w500:errorcluster, "pfPosition"=w495:sgl)  [unwired: 1 in, 2 out]
        "MirrorPosition" <- w495
        n196 = In Range and Coerce(upper limit=w533, x="Target Position", lower limit=w531) -> (coerced(x)=w535:dbl, In Range?=w534:bool)
        n197 = event shown="[2] \"Up\": Value Change" {
          selector: _ -> [_ _ _]
          dyn-events: _ -> [_ _ _]
          timeout: 1 -> [_ _ _]
          tunnel: "Up" -> [_ _ _]
          tunnel: "Down" -> [_ _ _]
          tunnel: 0.1 -> [_ w565 w569]
          tunnel: "Target Position" -> [_ w566 w568]
          event Timeout {
            n198 = event-data() -> ()  [unwired: 1 in, 2 out]
          }
          event "Down": Value Change {
            n199 = event-data() -> ()  [unwired: 1 in, 2 out]
            n200 = Subtract(x=w566, y=w565) -> (x-y=w564:dbl)
            n201 = local write "Target Position"(w564) -> ()
          }
          event "Up": Value Change {
            n202 = event-data() -> ()  [unwired: 1 in, 2 out]
            n203 = Add(x=w569, y=w568) -> (x+y=w567:dbl)
            n204 = local write "Target Position"(w567) -> ()
          }
        }
        n205 = feedback #2(w535) -> (w539:dbl)
        n206 = Not Equal?(x=w539, y=w535) -> (x != y?=w538:bool)
        n207 = feedback-in #2(w535) -> ()
        n208 = Or(x=w536, y=w538) -> (x .or. y?=w478:bool)
        n209 = case shown="True" "Home" {
          tunnel: w528 -> [w572 w578]
          tunnel: w515 -> [w571 w575]
          tunnel: [w572 w574] -> w527
          tunnel: [w571 w573] -> w526
          frame False {
          }
          frame True {
            n210 = invoke class="MG17Motor" method="MoveHome"(reference=w578, error in=w575, "lChanID"=0, "bWait"=FALSE) -> (reference out=w574:refnum<k7>, error out=w573:errorcluster)  [unwired: 1 in, 3 out]
          }
        }
        n211 = feedback #3(w495) -> (w499:sgl)
        n212 = Not Equal?(x=w495, y=w499) -> (x != y?=w477:bool)
        n213 = feedback-in #3(w495) -> ()
        n214 = Round To Nearest(number=w495) -> (nearest integer value=w456:sgl)
        n215 = local read "Old possition"() -> (w496:sgl)
        n216 = Not Equal?(x=w496, y=w456) -> (x != y?=w494:bool)
        n217 = Not Equal?(x=w456, y=w457) -> (x != y?=w455:bool)
        n218 = Or(x=w477, y=w478) -> (x .or. y?=w458:bool)
        "Moving" <- w458
        n219 = Not(x=w477) -> (.not. x?=w498:bool)
        n220 = And(x=w498, y=w494) -> (x .and. y?=w497:bool)
        n221 = Not(x=w534) -> (.not. x?=w459:bool)
        n222 = case shown="True" w497 {
          tunnel: w457 -> [_ w560]
          tunnel: ["Mirror\nOverride" TRUE] -> w493
          frame False {
          }
          frame True {
            "Old possition" <- w560
          }
        }
        n223 = Compound Arithmetic op=OR(w455, w458, w459) -> (→"Error/Wait":bool)
        n224 = case shown="True" w458 {
          tunnel: w527 -> [w579 w589]
          tunnel: w535 -> [_ w585]
          tunnel: w526 -> [w580 w584]
          tunnel: [w580 w582] -> w529
          tunnel: [w579 w581] -> w530
          frame False {
          }
          frame True {
            w586 = 0 ("lChanID")
            n225 = invoke class="MG17Motor" method="SetAbsMovePos"(reference=w589, error in=w584, "lChanID"=w586, "fAbsPos"=w585) -> (reference out=w588:refnum<k7>, error out=w583:errorcluster)  [unwired: 1 in, 3 out]
            n226 = invoke class="MG17Motor" method="MoveAbsolute"(reference=w588, error in=w583, "lChanID"=w586, "bWait"=FALSE) -> (reference out=w581:refnum<k7>, error out=w582:errorcluster)  [unwired: 1 in, 3 out]
          }
        }
        n227 = Build Array(w493) -> (w483:bool[])
        n228 = Compound Arithmetic op=OR("stop", w453) -> (w523:bool)
        n229 = call-poly <vilib>:"DAQmx Write.vi"("task/channels in"=w480, "data"=w483, "error in"=w479) -> ("task out"=w482:refnum<k21>, "error out"=w481:errorcluster)  [unwired: 10 in, 1 out]
      }
      frame "Read Calibration" {
        n230 = local read "SavePath"() -> (w592:path)
        n231 = Build Path(base path=w592, name or relative path=w610) -> (appended path=w599:path)
        n232 = shared-variable "My Computer\\Laser Library.lvlib\\WV"() -> (w591:dbl)  [unwired: 1 in, 1 out]
        n233 = local read "Scaner"() -> (w593:string)
        n234 = Build Path(base path=w599, name or relative path=w593) -> (appended path=w600:path)
        n235 = Number To Decimal String(number="Lens") -> (decimal integer string=w612:string)  [unwired: 1 in]
        n236 = Number To Decimal String(number=w591) -> (decimal integer string=w601:string)  [unwired: 1 in]
        n237 = Build Path(base path=w600, name or relative path=w612) -> (appended path=w596:path)
        n238 = shared-variable "My Computer\\Laser Library.lvlib\\GDD"() -> (w598:dbl)  [unwired: 1 in, 1 out]
        n239 = Concatenate Strings(w601, "\\" ("string")) -> (w607:string)
        n240 = Build Path(base path=w596, name or relative path=w607) -> (appended path=w595:path)
        n241 = Number To Decimal String(number=w598) -> (decimal integer string=w597:string)  [unwired: 1 in]
        n242 = shared-variable "My Computer\\Laser Library.lvlib\\Lens"("Lens") -> ()  [unwired: 1 in, 1 out]
        n243 = Build Path(base path=w595, name or relative path=w597) -> (appended path=w594:path)
        n244 = List Folder(path=w594) -> (filenames=w611:string[], error out=w606:errorcluster)  [unwired: 3 in, 2 out]
        n245 = Unbundle By Name(w606) -> ("status"=w603:bool)
        n246 = Array Size(array=w611) -> (size(s)=w609:i32)
        n247 = Not Equal To 0?(x=w609) -> (x != 0?=w604:bool)
        n248 = Not(x=w603) -> (.not. x?=w602:bool)
        n249 = And(x=w604, y=w602) -> (x .and. y?=w605:bool)
        n250 = case shown="False" w605 {
          tunnel: w611 -> [_ w640]
          tunnel: w609 -> [_ w639]
          tunnel: w594 -> [_ w637]
          tunnel: w591 -> [_ w622]
          frame False {
            n251 = local write "Power (mW)"(-1) -> ()
          }
          frame True {
            w628 = 2 items=["nearest", "linear", "spline", "cubic Hermite", "Lagrange"] ("method")
            n252 = feedback-in #4(w622) -> ()
            n253 = feedback #4() -> (w621:dbl)  [unwired: 1 in]
            n254 = Not Equal?(x=w622, y=w621) -> (x != y?=w618:bool)
            n255 = Decrement(x=w639) -> (x-1=w638:i32)
            n256 = flat-sequence "Select Position from commanded power" {
              tunnel: w624 -> [w668]
              tunnel: w623 -> [w657]
              tunnel: [w653] -> w620
              tunnel: w618 -> [w641]
              tunnel: [w641] -> w617
              tunnel: w620 -> [w679]
              tunnel: w619 -> [w676]
              tunnel: w617 -> [w675]
              frame #0 {
                w652 = 2 items=["nearest", "linear", "spline", "cubic Hermite", "Lagrange"] ("method")
                w664 = 0 items=["nearest", "linear", "spline", "cubic Hermite", "Lagrange"] ("method")
                n257 = local read "Power Min&Max"() -> (w663:i32[])
                n258 = Index Array(array=w663, index=1) -> (element=w644:i32)
                n259 = Index Array(array=w663, index=0) -> (element=w643:i32)
                n260 = Greater?(x=w657, y=w643) -> (0:w662:bool[])
                n261 = Greater?(x=w657, y=w644) -> (0:w659:bool[])
                n262 = Subtract(x=w644, y=w643) -> (x-y=w642:i32)
                n263 = Search 1D Array(1D array=w662, element=TRUE) -> (index of element=w660:i32)  [unwired: 1 in]
                n264 = Search 1D Array(1D array=w659, element=TRUE) -> (index of element=w656:i32)  [unwired: 1 in]
                n265 = Multiply(x=w642, y=10.0) -> (x*y=w645:dbl)
                n266 = Subtract(x=w656, y=w660) -> (x-y=w667:i32)
                n267 = for {
                  N: w645 -> [_]
                  tunnel: [w671] -> w649 mode=indexing
                  shift-right: [w671] -> _
                  shift-left: w643 -> [w672]
                  n268 = Add(x=0.1, y=w672) -> (x+y=w671:dbl)
                }
                n269 = Array Subset "Sub-positions"(array=w657, index=w660, length=w667) -> (w650:dbl[])
                n270 = Array Subset "Sub-Power"(array=w668, index=w660, length=w667) -> (w651:dbl[])
                n271 = local read "Power (mW)"() -> (w653:dbl)
                n272 = call <vilib>:"Interpolate 1D.vi"("method"=w652, "xi"=w649, "X"=w650, "Y"=w651) -> ("xi used"=w648:dbl[], "yi"=w647:dbl[])  [unwired: 5 in, 1 out]
                n273 = Build Array(w653) -> (w666:dbl[])
                n274 = call <vilib>:"Interpolate 1D.vi"("method"=w664, "xi"=w666, "X"=w647, "Y"=w648) -> ("yi"=w665:dbl[])  [unwired: 5 in, 2 out]
                n275 = Index Array(array=w665) -> (element=w655:dbl)  [unwired: 1 in]
                n276 = event shown="[1] \"Power (mW)\": Value Change" {
                  selector: _ -> [_ _]
                  dyn-events: _ -> [_ _]
                  timeout: 1 -> [_ _]
                  tunnel: w655 -> [_ w674]
                  event Timeout {
                    n277 = event-data() -> ()  [unwired: 1 in, 2 out]
                  }
                  event "Power (mW)": Value Change {
                    n278 = event-data() -> ()  [unwired: 1 in, 2 out]
                    n279 = local write "Target Position"(w674) -> ()
                  }
                }
              }
              frame #1 {
                n280 = And(x="Auto", y=w675) -> (x .and. y?=w678:bool)
                n281 = case shown="False" w678 {
                  tunnel: w679 -> [_ w681]
                  tunnel: w676 -> [w680 _]
                  frame False {
                    n282 = local write "Power (mW)"(w680) -> ()
                  }
                  frame True {
                    n283 = property on="Power (mW)" class="DigNum (strict)"("Val(Sgnl)"=w681) -> ()  [unwired: 2 in, 2 out]
                  }
                }
              }
            }
            n284 = Index Array(array=w640, index=w638) -> (element=w636:string)
            "Calibration Used" <- w636
            n285 = Build Path(base path=w637, name or relative path=w636) -> (appended path=w635:path)
            n286 = local read "Current Position"() -> (w634:sgl)
            n287 = call-poly <vilib>:"Read From Spreadsheet File.vi"("delimiter (\\t)"="," ("delimiter (\\t)"), "format (%.3f)"="%.6f", "file path (dialog if empty)"=w635) -> ("all rows"=w633:dbl[][])  [unwired: 4 in, 4 out]
            n288 = Build Array(w634) -> (w625:sgl[])
            n289 = Index Array "Power"(array=w633, index (row)=1 ("disabled index (col)")) -> (element=w624:dbl[])  [unwired: 1 in]
            n290 = Index Array "Position"(array=w633, index (row)=0 ("disabled index (col)")) -> (element=w623:dbl[])  [unwired: 1 in]
            n291 = Bundle("all rows"=w623, "all rows"=w624) -> (→"Curve":cluster{"all rows":dbl[], "all rows":dbl[]})  [unwired: 1 in]
            n292 = call <vilib>:"Interpolate 1D.vi"("method"=w628, "xi"=w625, "X"=w623, "Y"=w624) -> ("yi"=w627:dbl[])  [unwired: 5 in, 2 out]
            n293 = Index Array(array=w627) -> (element=w619:dbl)  [unwired: 1 in]
          }
        }
      }
    }
    n294 = Wait (ms)(milliseconds to wait=u32 50) -> ()  [unwired: 1 out]
  }
  n295 = call <vilib>:"DAQmx Stop Task.vi"("task/channels in"=w19, "error in"=w18) -> ()  [unwired: 12 in, 2 out]
  n296 = invoke class="MG17Motor" method="StopCtrl"(reference=w45, error in=w46) -> (error out=w44:errorcluster)  [unwired: 1 in, 2 out]
  n297 = invoke class="MG17Motor" method="StopCtrl"(reference=w25, error in=w24) -> (error out=w26:errorcluster)  [unwired: 1 in, 2 out]
  n298 = call <vilib>:"Clear Errors.vi"("error in (no error)"=w44) -> ()  [unwired: 5 in, 2 out]
  n299 = call <vilib>:"Clear Errors.vi"("error in (no error)"=w26) -> ()  [unwired: 5 in, 2 out]
  "SavePath" <- "Path"
